vi "OHM Range.vi"() -> ()   [LabVIEW 2020, in "Yokogawa GX Series.lvlib"]
uses:
  <instrlib>/Yokogawa GX Series/Yokogawa GX Series.lvlib
panel:
  in  "OHM Range":string="20ohm\n200ohm\n2000ohm"
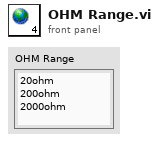
[diagram p1: front panel]
diagram:
